vi "testDemo2.vi"(8 "error in (no error)":errorcluster, 11 "MyFirstTest.lvclass in":refnum<class "MyFirstTest.lvclass">) -> (0 "error out":errorcluster, 3 "MyFirstTest.lvclass out":refnum<class "MyFirstTest.lvclass">)   [LabVIEW 2011, in "MyFirstTest.lvclass"]
doc: "This VI is a demo test -- it ensures that \"dog\" != \"cat\""
uses:
  MyFirstTest.lvclass
panel:
  # "Copyright © 2007 James Kring, Inc. All rights reserved.\n\nAuthor: Jim Kring [jim.kring@jameskring.com]\n\nThis library is provided \"AS IS\" ,WITHOUT WARRANTIES OR \nCONDITIONS OF ANY KIND, either express or implied.\n\nJames Kring, Inc. -- http://www.jameskring.com"
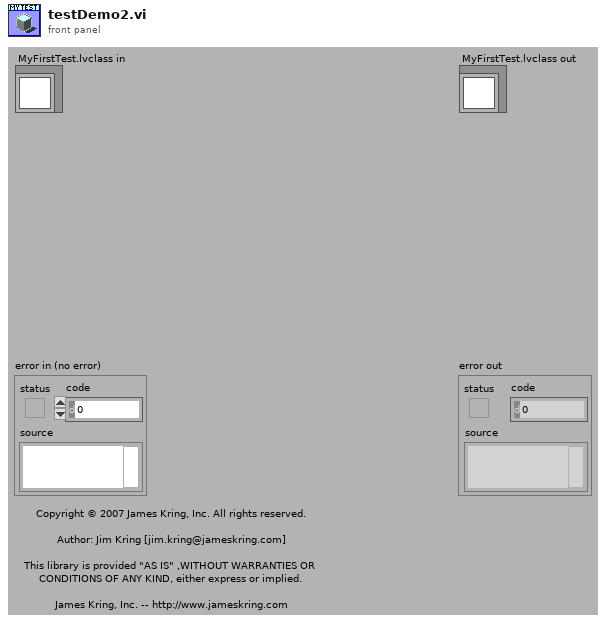
[diagram p1: front panel]
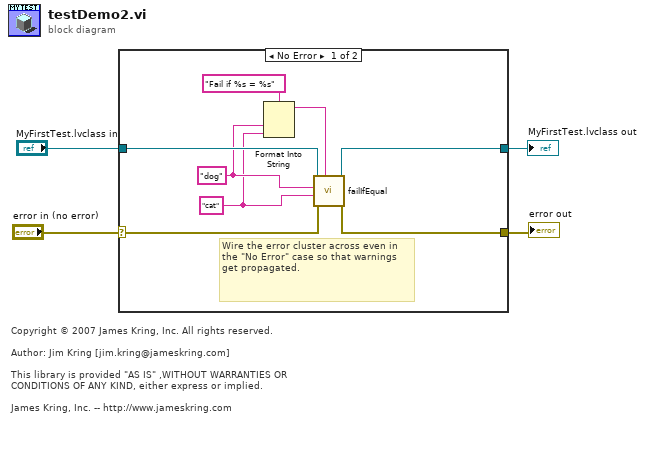
[diagram p0: block diagram]
diagram:
  # "Copyright © 2007 James Kring, Inc. All rights reserved.\n\nAuthor: Jim Kring [jim.kring@jameskring.com]\n\nThis library is provided \"AS IS\" ,WITHOUT WARRANTIES OR \nCONDITIONS OF ANY KIND, either express or implied.\n\nJames Kring, Inc. -- http://www.jameskring.com"
  n1 = case shown="No Error" "error in (no error)" {
    selector: "error in (no error)" -> [w10 w14]
    tunnel: [w9 w14] -> w3
    tunnel: [w11 w13] -> w1
    tunnel: "MyFirstTest.lvclass in" -> [w12 w13]
    frame No Error {
      w6 = "cat"
      w7 = "dog"
      # "Wire the error cluster across even in the \"No Error\" case so that warnings get propagated."
      n2 = Format Into String(format string="Fail if %s = %s", w7, w6) -> (resulting string=w5:string)  [unwired: 2 in, 1 out]
      n3 = call-dynamic "failIfEqual.vi"("custom report message (\"\")"=w5, "error in (no error)"=w10, "y"=w6, "x"=w7, "TestCase in"=w12) -> ("error out"=w9:errorcluster, "TestCase out"=w11:refnum<class "MyFirstTest.lvclass">)  [unwired: 5 in]
    }
    frame Error {
    }
  }
  "error out" <- w3
  "MyFirstTest.lvclass out" <- w1
